vi "Read Fast Tree.vi"(8 "error in":errorcluster, 11 "ParseGDSII in":refnum<class "ParseGDSII.lvclass">) -> (0 "error out":errorcluster, 1 "Fast Tree.lvclass":refnum<class "Fast Tree.lvclass">, 2 "Tree":T1(array[cluster]), 3 "ParseGDSII out":refnum<class "ParseGDSII.lvclass">)   [LabVIEW 2019, in "ParseGDSII.lvclass"]
uses:
  ParseGDSII.lvclass
  Fast Tree/Fast Tree.lvclass
  ParseGDSII.lvclass/ParseGDSII.ctl
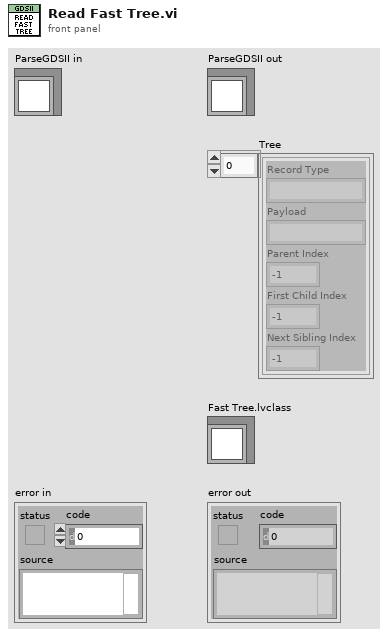
[diagram p1: front panel]
types:
  T1 = cluster{"Record Type":string, "Payload":string, "Parent Index":i32, "First Child Index":i32, "Next Sibling Index":i32}[]
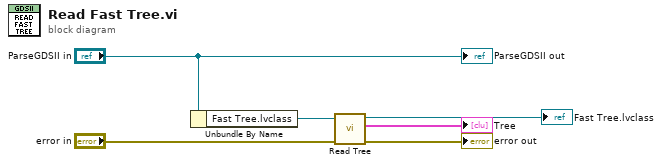
[diagram p0: block diagram]
diagram:
  n1 = Unbundle By Name("ParseGDSII in") -> ("Fast Tree.lvclass"=w6:refnum<class "Fast Tree.lvclass">)
  n2 = call-dynamic "Read Tree.vi"("error in (no error)"="error in", "Fast Tree in"=w6) -> ("error out"=→"error out":errorcluster, "Tree"=→"Tree":T1, "Fast Tree out"=→"Fast Tree.lvclass":refnum<class "Fast Tree.lvclass">)  [unwired: 7 in]
  "ParseGDSII out" <- "ParseGDSII in"
